vi "save_comments.vi"(8 "error in":errorcluster, 10 "Str Refnum":refnum<vi>, 11 "base path":path) -> (0 "error out":errorcluster)   [LabVIEW 2013]
panel:
  in  "Continue":bool
  in  "Please complete the notes for this experiment.  Then click":string
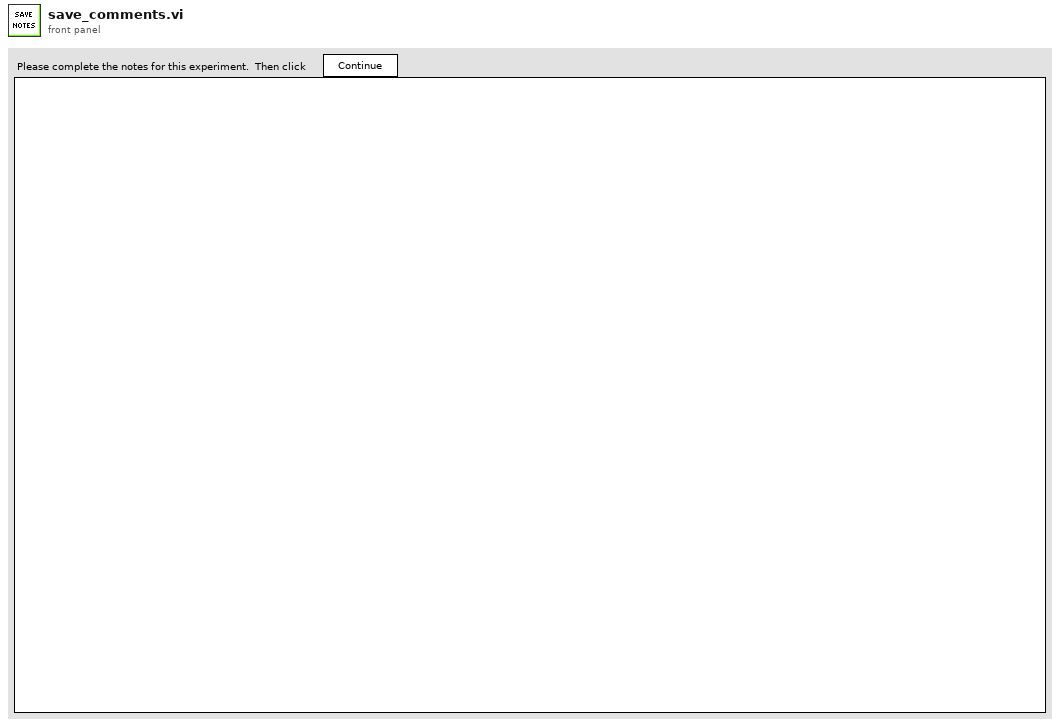
[diagram p1: front panel]
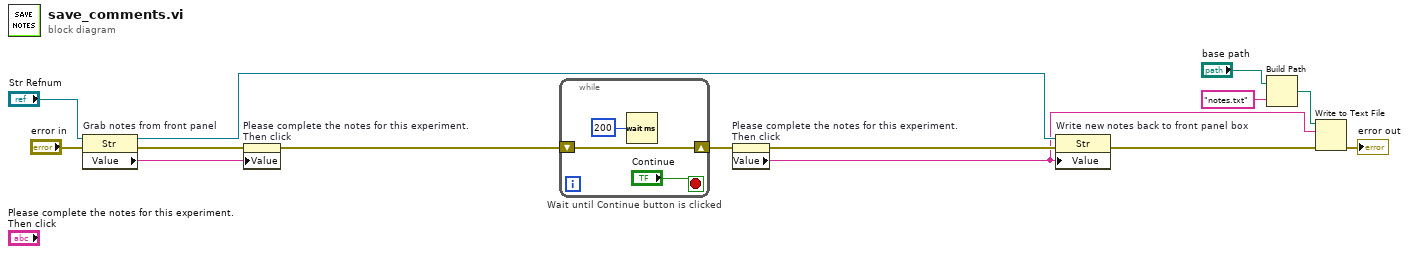
[diagram p0: block diagram]
diagram:
  n1 = property on="Grab notes from front panel" class="Str"(reference="Str Refnum", error in="error in") -> (reference out=w2:refnum<vi>, error out=w7:errorcluster, "Value"=w8:string)
  n2 = property on="Please complete the notes for this experiment.  Then click" class="Str"(error in=w7, "Value"=w8) -> (error out=w5:errorcluster)  [unwired: 1 in, 1 out]
  n3 = while "Wait until Continue button is clicked" {
    shift-right: [w16] -> w10
    shift-left: w5 -> [w16]
    stop <- "Continue" stop-if-true
    n4 = Wait (ms)(milliseconds to wait=u32 200) -> ()  [unwired: 1 out]
  }
  n5 = property on="Please complete the notes for this experiment.  Then click" class="Str"(error in=w10) -> (error out=w4:errorcluster, "Value"=w1:string)  [unwired: 1 in, 1 out]
  n6 = property on="Write new notes back to front panel box" class="Str"(reference=w2, error in=w4, "Value"=w1) -> (error out=w3:errorcluster)  [unwired: 1 out]
  n7 = Build Path(base path="base path", name or relative path="notes.txt") -> (appended path=w12:path)
  n8 = Write to Text File(file (use dialog)=w12, text=w1, error in=w3) -> (error out=→"error out":errorcluster)  [unwired: 1 in, 2 out]
